vi "Teleop.vi"(10 "Match Info":T1={"Autonomous Elapsed Seconds"=0.0, "TeleOp Elapsed Seconds"=0.0, "Disabled Elapsed Seconds"=0.0, "Visited Autonomous"=FALSE, "Visited TeleOp"=FALSE, "Visited Disabled"=FALSE, "Autonomous Settings"={"Autonomous Style"=enum."Independent", "VI Refnum"=refnum}}, 11 "Call Context":T2) -> ()   [LabVIEW 2018]
doc: "This VI is called for each TeleOp packet received from the DS where the robot is not disabled. It is often used to read from the joysticks and update I/O or to update setpoints for timed control loops. It should complete and return within 20 milliseconds or it may miss DS packets."
uses:
  <vilib>/Rock Robotics/WPI/DriverStation/WPI_DriverStationDerivedRobotMode.ctl
  <vilib>/Rock Robotics/WPI/DriverStation/WPI_DriverStationMatch Info.ctl
  <vilib>/Rock Robotics/WPI/Solenoid/WPI_SolenoidValue.ctl
  <vilib>/Rock Robotics/WPI/Utilities/WPI_GetSetVariantRefNum.vi
  <vilib>/Rock Robotics/Network Tables/NT Write Boolean Array.vi
  <vilib>/Rock Robotics/Network Tables/NT Write Numeric Array.vi
  <vilib>/Rock Robotics/Network Tables/NT Read Boolean.vi
  <vilib>/Rock Robotics/Network Tables/NT Read Number.vi
  Robot Global Data.vi
  <vilib>/Rock Robotics/Network Tables/NT Write Number.vi
  <vilib>/Rock Robotics/WPI/Solenoid/WPI_SolenoidSetEnum.vi
panel:
  out "Sample Slider 0":dbl(slide) scale=0.0..5.0
  out "Sample Boolean 1":bool
  out "Sample Boolean 0":bool
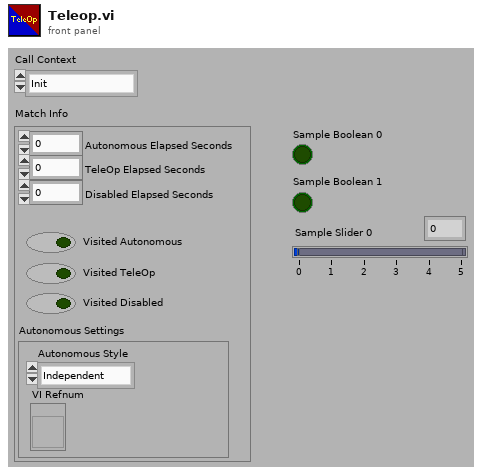
[diagram p1: front panel]
types:
  T1 = typedef "WPI_DriverStationMatch Info.ctl" = cluster{"Autonomous Elapsed Seconds":dbl, "TeleOp Elapsed Seconds":dbl, "Disabled Elapsed Seconds":dbl, "Visited Autonomous":bool, "Visited TeleOp":bool, "Visited Disabled":bool, "Autonomous Settings":cluster{"Autonomous Style":enum16{"Iterative", "Independent"}, "VI Refnum":refnum<vi>}}
  T2 = typedef "WPI_DriverStationDerivedRobotMode.ctl" = enum16{"Init", "Execute", "Stop"}
  T3 = typedef "WPI_SolenoidValue.ctl" = enum16{"Off", "On", "Forward", "Reverse"}
  T4 = typedef "WPI_RobotDriveDevRef.ctl" = cluster{"DevStatus":errorcluster, "Motors[]":T5[], "Square Inputs":bool, "Max Output":dbl}
  T5 = typedef "WPI_MotorControlDeviceRef.ctl" = cluster{"DeviceStatus":errorcluster, "Type":T6, "PWM":cluster{"PWM Channel":T7, "DeadBand":T8}, "CAN":cluster{"Device Number":u8, "SetOutput VI Ref":variant, "GetOutput VI Ref":variant, "Enable VI Ref":variant, "Disable VI Ref":variant, "Data":variant}, "Invert":bool, "DIO PWM":cluster{"PWM \"Enable\" Channel":T7, "DIOChannel":T9, "PWM Rate":dbl}}
  T6 = typedef "WPI_MotorControlType.ctl" = enum16{"PWM", "CAN", "DIO PWM"}
  T7 = typedef "FPGA_DIOPWMChannel.ctl" = enum8{"PWM 0", "PWM 1", "PWM 2", "PWM 3", "PWM 4", "PWM 5", "PWM 6", "PWM 7", "PWM 8", "PWM 9", "PWM MXP 0", "PWM MXP 1", "PWM MXP 2", "PWM MXP 3", "PWM MXP 4", "PWM MXP 5", "PWM MXP 6", "PWM MXP 7", "PWM MXP 8", "PWM MXP 9", "Invalid"}
  T8 = typedef "WPI_PWMDeadband.ctl" = cluster{"Name":string, "maxPositivePwm":i32, "minPositivePwm":i32, "centerPwm":i32, "maxNegativePwm":i32, "minNegativePwm":i32, "angularRange":u16}
  T9 = typedef "FPGA_DIOChannel.ctl" = enum8{"DIO 0", "DIO 1", "DIO 2", "DIO 3", "DIO 4", "DIO 5", "DIO 6", "DIO 7", "DIO 8", "DIO 9", "DIO MXP 0", "DIO MXP 1", "DIO MXP 2", "DIO MXP 3", "DIO MXP 4", "DIO MXP 5", "DIO MXP 6", "DIO MXP 7", "DIO MXP 8", "DIO MXP 9", "DIO MXP 10", "DIO MXP 11", "DIO MXP 12", "DIO MXP 13", "DIO MXP 14", "DIO MXP 15", "SPI Port CS1", "SPI Port CS2", "SPI Port CS3", "SPI Port MISO", "SPI Port MOSI", "Invalid"}
  T10 = typedef "WPI_JoystickDevRef.ctl" = cluster{"Device":T11}
  T11 = typedef "WPI_JoystickDeviceEnum.ctl" = enum16{"USB 0", "USB 1", "USB 2", "USB 3", "USB 4", "USB 5"}
  T12 = typedef "WPI_EncoderDevRef.ctl" = cluster{"DevStatus":errorcluster, "EncoderIndex":T13, "CounterIndex":T14, "DistancePerCount":dbl, "Decoding Type":T15}
  T13 = typedef "FPGA_EncoderIdx.ctl" = enum8{"Enc 0", "Enc 1", "Enc 2", "Enc 3", "Enc 4", "Enc 5", "Enc 6", "Enc 7", "Invalid"}
  T14 = typedef "FPGA_CounterCtrSystemIndex.ctl" = enum8{"Ctr 0", "Ctr 1", "Ctr 2", "Ctr 3", "Ctr 4", "Ctr 5", "Ctr 6", "Ctr 7", "Invalid"}
  T15 = typedef "WPI_EncoderType.ctl" = enum16{"1x", "2x", "4x"}
  T16 = typedef "WPI_SolenoidDevRef.ctl" = cluster{"DevStatus":errorcluster, "Pneumatics Control Module":u8, "Forward Solenoid Channel":T17, "Reverse Solenoid Channel":T17}
  T17 = typedef "WPI_SolenoidChannel.ctl" = enum8{"Solenoid 0", "Solenoid 1", "Solenoid 2", "Solenoid 3", "Solenoid 4", "Solenoid 5", "Solenoid 6", "Solenoid 7", "Invalid"}
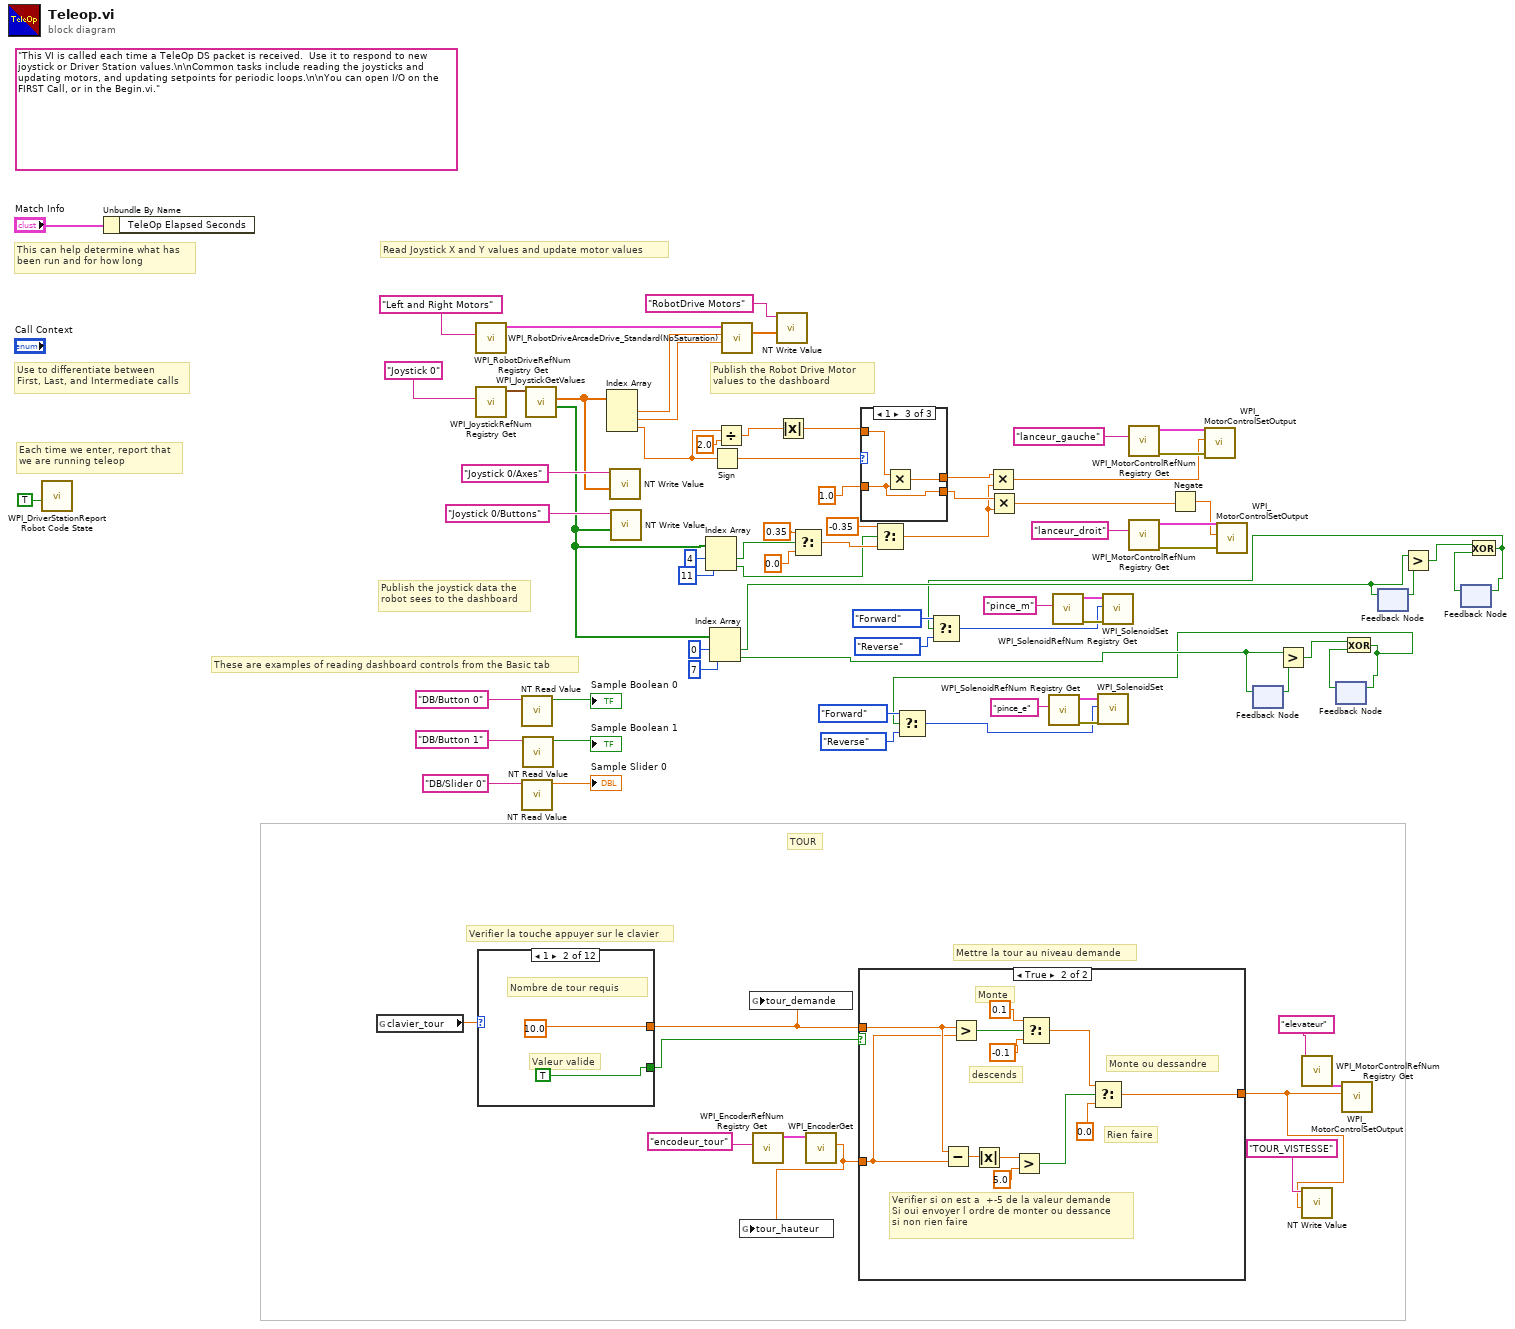
[diagram p0: block diagram]
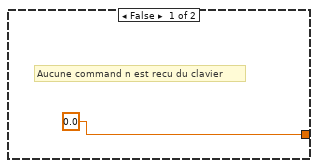
[diagram p2: hidden frame]
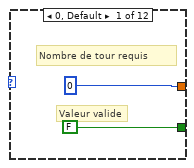
[diagram p3: hidden frame]
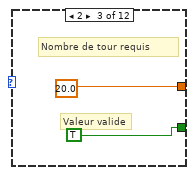
[diagram p4: hidden frame]
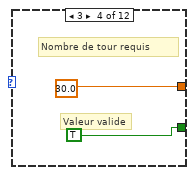
[diagram p5: hidden frame]
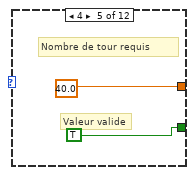
[diagram p6: hidden frame]
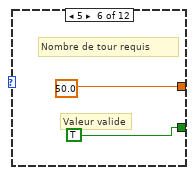
[diagram p7: hidden frame]
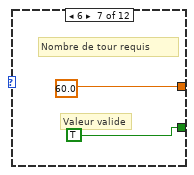
[diagram p8: hidden frame]
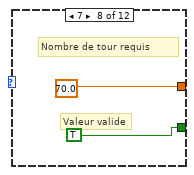
[diagram p9: hidden frame]
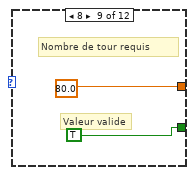
[diagram p10: hidden frame]
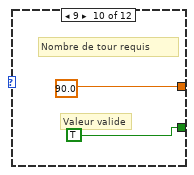
[diagram p11: hidden frame]
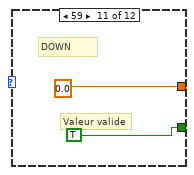
[diagram p12: hidden frame]
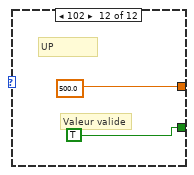
[diagram p13: hidden frame]
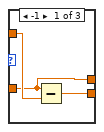
[diagram p14: hidden frame]
diagram:
  (unwired) "This VI is called each time a TeleOp DS packet is received.  Use it to respond to new joystick or Driver Station values.\n\nCommon tasks include reading the joysticks and updating motors, and updating setpoints for periodic loops.\n\nYou can open I/O on the FIRST Call, or in the Begin.vi."
  # "TOUR"
  # "Mettre la tour au niveau demande"
  # "Verifier la touche appuyer sur le clavier"
  # "These are examples of reading dashboard controls from the Basic tab"
  # "Publish the Robot Drive Motor\nvalues to the dashboard"
  # "Publish the joystick data the\nrobot sees to the dashboard"
  # "Each time we enter, report that\nwe are running teleop"
  # "Use to differentiate between\nFirst, Last, and Intermediate calls"
  # "This can help determine what has\nbeen run and for how long"
  # "Read Joystick X and Y values and update motor values"
  n1 = call <vilib>:"WPI_DriverStationReport Robot Code State.vi"("TeleOp"=TRUE ("Autonomous")) -> ()  [unwired: 10 in, 1 out]
  n2 = Unbundle By Name("Match Info") -> ()  [unwired: 1 out]
  n3 = global read "Robot Global Data.vi" "clavier_tour"() -> (w35:dbl)
  n4 = call <vilib>:"WPI_RobotDriveRefNum Registry Get.vi"("refnum name"="Left and Right Motors") -> ("RobotDriveDevRef"=w78:T4)  [unwired: 1 in, 9 out]
  n5 = call <vilib>:"WPI_JoystickRefNum Registry Get.vi"("refnum name"="Joystick 0") -> ("JoystickDevRef"=w75:T10)  [unwired: 1 in, 9 out]
  n6 = case shown="1" w35 {
    tunnel: [0 10.0 20.0 30.0 40.0 50.0 60.0 70.0 80.0 90.0 0.0 500.0] -> w34
    tunnel: [FALSE TRUE TRUE TRUE TRUE TRUE TRUE TRUE TRUE TRUE TRUE TRUE] -> w39
    frame 0, Default {
      # "Valeur valide"
      # "Nombre de tour requis"
    }
    frame 1 {
      # "Valeur valide"
      # "Nombre de tour requis"
    }
    frame 2 {
      # "Valeur valide"
      # "Nombre de tour requis"
    }
    frame 3 {
      # "Valeur valide"
      # "Nombre de tour requis"
    }
    frame 4 {
      # "Valeur valide"
      # "Nombre de tour requis"
    }
    frame 5 {
      # "Valeur valide"
      # "Nombre de tour requis"
    }
    frame 6 {
      # "Valeur valide"
      # "Nombre de tour requis"
    }
    frame 7 {
      # "Valeur valide"
      # "Nombre de tour requis"
    }
    frame 8 {
      # "Valeur valide"
      # "Nombre de tour requis"
    }
    frame 9 {
      # "Valeur valide"
      # "Nombre de tour requis"
    }
    frame 59 {
      # "Valeur valide"
      # "DOWN"
    }
    frame 102 {
      # "Valeur valide"
      # "UP"
    }
  }
  n7 = call-poly <vilib>:"NT Read Value.vi"("Name"="DB/Button 0" ("refnum name")) -> ("Boolean"=→"Sample Boolean 0":bool)  [unwired: 9 in, 1 out]
  n8 = call-poly <vilib>:"NT Read Value.vi"("Name"="DB/Slider 0" ("refnum name")) -> ("Numeric"=→"Sample Slider 0":dbl)  [unwired: 9 in, 1 out]
  n9 = call-poly <vilib>:"NT Read Value.vi"("Name"="DB/Button 1" ("refnum name")) -> ("Boolean"=→"Sample Boolean 1":bool)  [unwired: 9 in, 1 out]
  n10 = call <vilib>:"WPI_JoystickGetValues.vi"("JoystickDevRef"=w75) -> ("Buttons"=w50:bool[], "Axes"=w70:dbl[])  [unwired: 6 in, 3 out]
  n11 = Index Array(array=w70) -> (element #1=w77:dbl, element #2=w73:dbl, element #3=w29:dbl)  [unwired: 3 in]
  n12 = call-poly <vilib>:"NT Write Value.vi"("Numeric Array"=w70, "Name"="Joystick 0/Axes") -> ()  [unwired: 9 in, 1 out]
  n13 = call-poly <vilib>:"NT Write Value.vi"("Boolean Array"=w50, "Name"="Joystick 0/Buttons") -> ()  [unwired: 9 in, 1 out]
  n14 = Index Array(array=w50, index #1=4 ("index"), index #2=11 ("index")) -> (element #1=w56:bool, element #2=w26:bool)
  n15 = Index Array(array=w50, index #1=0 ("index"), index #2=7 ("index")) -> (element #1=w6:bool, element #2=w11:bool)
  n16 = Sign(1:w29) -> (0:w41:dbl)
  n17 = Divide(x=w29, y=2.0) -> (x/y=w30:dbl)
  n18 = call <vilib>:"WPI_RobotDriveArcadeDrive_Standard(NoSaturation).vi"("Y axis value"=w73, "X axis value"=w77, "RobotDriveDevRef"=w78) -> ("Motor Values"=w63:dbl[])  [unwired: 1 in, 7 out]
  n19 = global write "Robot Global Data.vi" "tour_demande"(w34) -> ()
  n20 = call <vilib>:"WPI_EncoderRefNum Registry Get.vi"("refnum name"="encodeur_tour" ("Name")) -> ("EncoderDevRef"=w37:T12)  [unwired: 9 in, 1 out]
  n21 = call-poly <vilib>:"NT Write Value.vi"("Numeric Array"=w63, "Name"="RobotDrive Motors") -> ()  [unwired: 9 in, 1 out]
  n22 = Absolute Value(x=w30) -> (abs(x)=w31:dbl)
  n23 = Select(t=0.35, s=w56, f=0.0) -> (s? t:f=w27:dbl)
  n24 = call <vilib>:"WPI_EncoderGet.vi"("EncoderDevRef"=w37) -> ("Distance"=w33:dbl)  [unwired: 5 in, 5 out]
  n25 = global write "Robot Global Data.vi" "tour_hauteur"(w33) -> ()
  n26 = case shown="True" w39 {
    tunnel: w34 -> [_ w114]
    tunnel: [0.0 w107] -> w2
    tunnel: w33 -> [_ w106]
    frame False {
      # "Aucune command n est recu du clavier"
    }
    frame True {
      # "Monte ou dessandre"
      # "Rien faire"
      # "Verifier si on est a  +-5 de la valeur demande\nSi oui envoyer l ordre de monter ou dessance \nsi non rien faire"
      # "descends"
      # "Monte"
      n27 = Subtract(x=w114, y=w106) -> (x-y=w113:dbl)
      n28 = Greater?(x=w114, y=w106) -> (0:w117:bool)
      n29 = Absolute Value(x=w113) -> (abs(x)=w112:dbl)
      n30 = Greater?(x=w112, y=5.0) -> (0:w110:bool)
      n31 = Select(t=0.1, s=w117, f=-0.1) -> (s? t:f=w109:dbl)
      n32 = Select(t=w109, s=w110, f=0.0) -> (s? t:f=w107:dbl)
    }
  }
  n33 = case shown="1" w41 {
    tunnel: [w118 w121 w124] -> w24
    tunnel: [w120 w121 w122] -> w23
    tunnel: w31 -> [w119 _ w123]
    tunnel: 1.0 -> [w118 w121 w122]
    frame -1 {
      n34 = Subtract(x=w118, y=w119) -> (x-y=w120:dbl)
    }
    frame 0, Default {
    }
    frame 1 {
      n35 = Multiply(x=w123, y=w122) -> (x*y=w124:dbl)
    }
  }
  n36 = Select(t=-0.35, s=w26, f=w27) -> (s? t:f=w20:dbl)
  n37 = Multiply(x=w24, y=w20) -> (x*y=w22:dbl)
  n38 = Multiply(x=w23, y=w20) -> (x*y=w21:dbl)
  n39 = call <vilib>:"WPI_SolenoidRefNum Registry Get.vi"("refnum name"="pince_e") -> ("error out"=w42:errorcluster, "SolenoidDevRef"=w43:T16)  [unwired: 9 in]
  n40 = call <vilib>:"WPI_SolenoidRefNum Registry Get.vi"("refnum name"="pince_m") -> ("error out"=w45:errorcluster, "SolenoidDevRef"=w44:T16)  [unwired: 9 in]
  n41 = call <vilib>:"WPI_MotorControlRefNum Registry Get.vi"("refnum name"="lanceur_gauche") -> ("error out"=w59:errorcluster, "MotorControlDevRef"=w53:T5)  [unwired: 9 in]
  n42 = call <vilib>:"WPI_MotorControlRefNum Registry Get.vi"("refnum name"="lanceur_droit") -> ("error out"=w57:errorcluster, "MotorControlDevRef"=w58:T5)  [unwired: 9 in]
  n43 = Negate(x=w21) -> (-x=w54:dbl)
  n44 = call <vilib>:"WPI_MotorControlSetOutput.vi"("error in (no error)"=w59, "Output"=w22, "MotorControlDevRef"=w53) -> ()  [unwired: 6 in, 3 out]
  n45 = call <vilib>:"WPI_MotorControlSetOutput.vi"("error in (no error)"=w57, "Output"=w54, "MotorControlDevRef"=w58) -> ()  [unwired: 6 in, 3 out]
  n46 = feedback #1() -> (w10:bool)  [unwired: 1 in]
  n47 = feedback-in #1(w11) -> ()
  n48 = Greater?(x=w11, y=w10) -> (0:w13:bool)
  n49 = call <vilib>:"WPI_MotorControlRefNum Registry Get.vi"("refnum name"="elevateur") -> ("MotorControlDevRef"=w38:T5)  [unwired: 9 in, 1 out]
  n50 = call-poly <vilib>:"NT Write Value.vi"("Numeric"=w2, "Name"="TOUR_VISTESSE") -> ()  [unwired: 9 in, 1 out]
  n51 = feedback #2() -> (w12:bool)  [unwired: 1 in]
  n52 = call <vilib>:"WPI_MotorControlSetOutput.vi"("Output"=w2, "MotorControlDevRef"=w38) -> ()  [unwired: 7 in, 3 out]
  n53 = Exclusive Or(1:w12, 2:w13) -> (0:w9:bool)
  n54 = Select(t=WPI_SolenoidValue."Forward" ("Value"), s=w9, f=WPI_SolenoidValue."Reverse" ("Value")) -> (s? t:f=w14:T3)
  n55 = call-poly <vilib>:"WPI_SolenoidSet.vi"("error in (no error)"=w42, "Value"=w14, "SolenoidDevRef"=w43) -> ()  [unwired: 7 in, 2 out]
  n56 = feedback-in #2(w9) -> ()
  n57 = feedback #3() -> (w5:bool)  [unwired: 1 in]
  n58 = feedback-in #3(w6) -> ()
  n59 = Greater?(x=w6, y=w5) -> (0:w8:bool)
  n60 = feedback #4() -> (w7:bool)  [unwired: 1 in]
  n61 = Exclusive Or(1:w7, 2:w8) -> (0:w4:bool)
  n62 = Select(t=WPI_SolenoidValue."Forward" ("Value"), s=w4, f=WPI_SolenoidValue."Reverse" ("Value")) -> (s? t:f=w15:T3)
  n63 = call-poly <vilib>:"WPI_SolenoidSet.vi"("error in (no error)"=w45, "Value"=w15, "SolenoidDevRef"=w44) -> ()  [unwired: 7 in, 2 out]
  n64 = feedback-in #4(w4) -> ()
